vi "Sound Test.vi"() -> ()   [LabVIEW 2009]
panel:
  out "name 5":string
  out "stripped path 5":path
  out "name 4":string
  out "stripped path 4":path
  out "name 3":string
  out "stripped path 3":path
  out "name 2":string
  out "stripped path 2":path
  out "stripped path":path
  out "name":string
  out "path":path
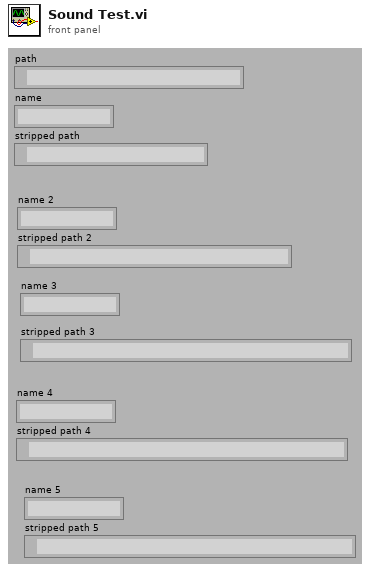
[diagram p1: front panel]
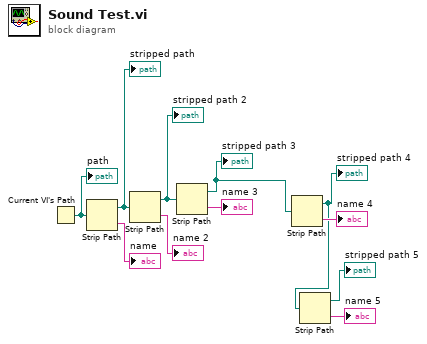
[diagram p0: block diagram]
diagram:
  n1 = Current VI's Path() -> (path=w8:path)
  "path" <- w8
  n2 = Strip Path(path=w8) -> (stripped path=w7:path, name=→"name":string)
  "stripped path" <- w7
  n3 = Strip Path(path=w7) -> (stripped path=w6:path, name=→"name 2":string)
  "stripped path 2" <- w6
  n4 = Strip Path(path=w6) -> (stripped path=w4:path, name=→"name 3":string)
  "stripped path 3" <- w4
  n5 = Strip Path(path=w4) -> (stripped path=w1:path, name=→"name 4":string)
  "stripped path 4" <- w1
  n6 = Strip Path(path=w1) -> (stripped path=→"stripped path 5":path, name=→"name 5":string)
